vi "Frequency Glide.vi"(5 "Fend (Hz)":dbl=2000.0, 7 "Fs (Hz)":dbl=100000.0, 9 "Npts":i32) -> (6 "Y":dbl[](array[numeric]))   [LabVIEW 2015]
uses:
  <vilib>/Analysis/1siggen.llb/Ramp Pattern by Samples.vi
  <vilib>/Analysis/NI_AALBase.lvlib
panel:
  in  "reset signal":bool
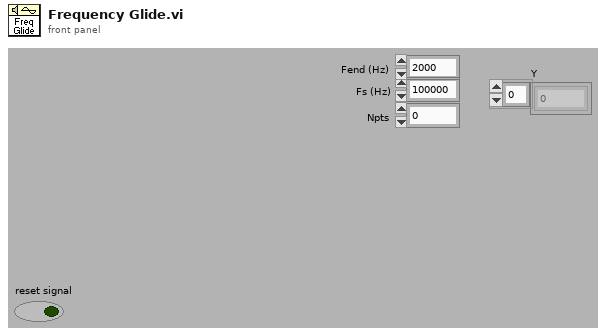
[diagram p1: front panel]
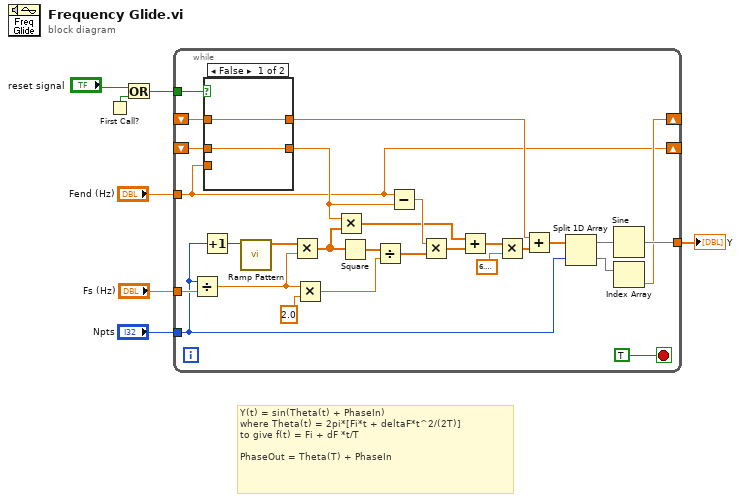
[diagram p0: block diagram]
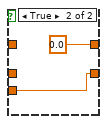
[diagram p2: hidden frame]
diagram:
  # "Y(t) = sin(Theta(t) + PhaseIn)\nwhere Theta(t) = 2pi*[Fi*t + deltaF*t^2/(2T)]\nto give f(t) = Fi + dF *t/T \n\nPhaseOut = Theta(T) + PhaseIn"
  n1 = First Call?() -> (First Call?: T/F=w2:bool)
  n2 = Or(x="reset signal", y=w2) -> (x .or. y?=w1:bool)
  n3 = while {
    tunnel: "Fs (Hz)" -> [w35]
    tunnel: "Npts" -> [w16]
    tunnel: "Fend (Hz)" -> [w8]
    tunnel: [w23] -> w4
    tunnel: w1 -> [w13]
    shift-right: [w14] -> _
    shift-left: _ -> [w12]
    shift-right: [w8] -> _
    shift-left: _ -> [w10]
    stop <- TRUE stop-if-true
    n4 = Divide(x=w16, y=w35) -> (x/y=w25:dbl)
    n5 = Increment(x=w16) -> (x+1=w20:i32)
    n6 = case shown="False" w13 {
      tunnel: w12 -> [w37 _]
      tunnel: [w37 0.0] -> w11
      tunnel: w10 -> [w36 _]
      tunnel: [w36 w38] -> w9
      tunnel: w8 -> [_ w38]
      frame False {
      }
      frame True {
      }
    }
    n7 = call-poly <vilib>:"Ramp Pattern.vi"("samples"=w20) -> ("Ramp Pattern"=w34:dbl[])  [unwired: 9 in, 1 out]
    n8 = Multiply(x=w34, y=w25) -> (x*y=w24:dbl[])
    n9 = Multiply(x=w25, y=2.0) -> (x*y=w31:dbl)
    n10 = Multiply(x=w9, y=w24) -> (x*y=w21:dbl[])
    n11 = Square(x=w24) -> (x^2=w32:dbl[])
    n12 = Divide(x=w32, y=w31) -> (x/y=w29:dbl[])
    n13 = Subtract(x=w8, y=w9) -> (x-y=w30:dbl)
    n14 = Multiply(x=w30, y=w29) -> (x*y=w28:dbl[])
    n15 = Add(x=w21, y=w28) -> (x+y=w22:dbl[])
    n16 = Multiply(x=w22, y=6.283185307179586) -> (x*y=w26:dbl[])
    n17 = Add(x=w11, y=w26) -> (x+y=w18:dbl[])
    n18 = Split 1D Array(array=w18, index=w16) -> (first subarray=w17:dbl[], second subarray=w15:dbl[])
    n19 = Sine(x=w17) -> (sin(x)=w23:dbl[])
    n20 = Index Array(array=w15) -> (element=w14:dbl)  [unwired: 1 in]
  }
  "Y" <- w4
